vi "Init.vi"(8 "error in (no error)":errorcluster, 9 "Config Fields":T1[](array[typedef]), 10 "Task Type":string, 11 "Name":string) -> (0 "error out":errorcluster, 3 "Task Config out":refnum<class "Task Config.lvclass">)   [LabVIEW 2020, in "Vecto.lvlib" / "Task Config.lvclass"]
uses:
  Task Config.lvclass
  Config Pair.ctl
  Vecto.lvlib
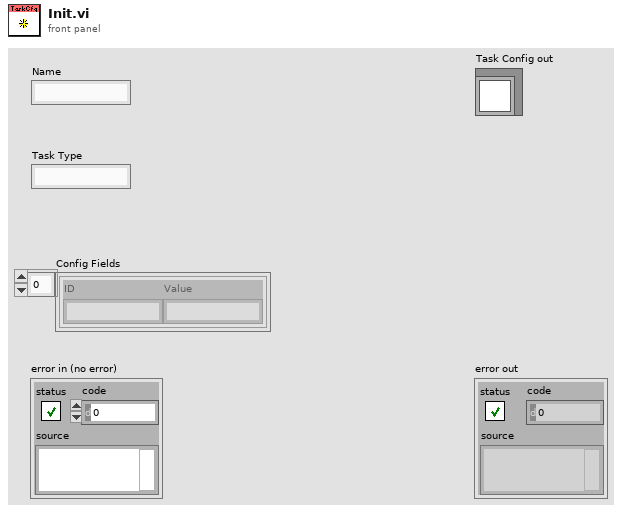
[diagram p1: front panel]
types:
  T1 = typedef "Vecto.lvlib/Config Pair.ctl" = cluster{"ID":string, "Value":string}
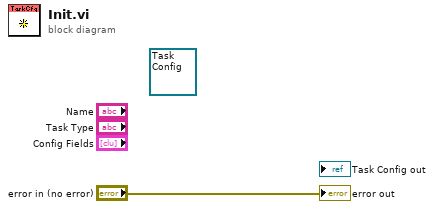
[diagram p0: block diagram]
diagram:
  (unwired) refnum<class "Task Config.lvclass"> refnum ("Task Config in")
  "error out" <- "error in (no error)"
